vi "sv_Flat Pink Noise Filter Coefficients.vi"() -> (1 "pink noise coeffs out":T1[](array[typedef]) {"order" format="%#_6p"})   [LabVIEW 2017]
uses:
  <vilib>/addons/_NISVFA/_Generation/subVIs/sv_Flat Pink Noise Coefficients.ctl
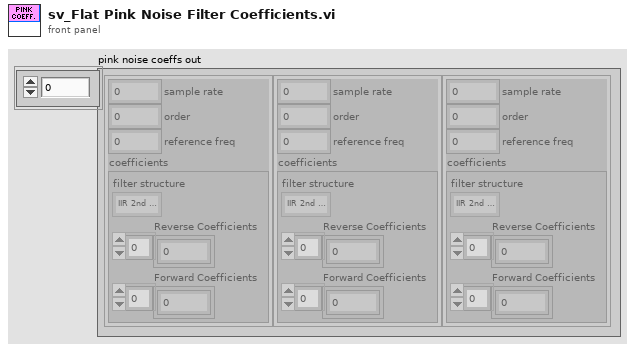
[diagram p1: front panel]
types:
  T1 = typedef "sv_Flat Pink Noise Coefficients.ctl" = cluster{"sample rate":dbl, "order":i32, "reference freq":dbl, "coefficients":cluster{"filter structure":enum32{"IIR 2nd Order", "IIR 4th Order"}, "Reverse Coefficients":dbl[], "Forward Coefficients":dbl[]}}
  T2 = cluster{"filter structure":enum32{"IIR 2nd Order", "IIR 4th Order"}, "b[i]":dbl[], "b[i]":dbl[]}
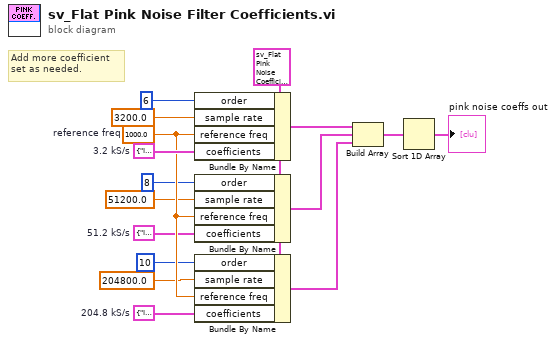
[diagram p0: block diagram]
diagram:
  w2 = T1 {"sample rate"=0.0, "order"=0, "reference freq"=0.0, "coefficients"={"filter structure"=enum."IIR 2nd Order", "Reverse Coefficients"=[-0.7577817918160894, 0.030536312542661648, -1.9301693255314603, 0.9308166907598192, -1.9976993495401576, 0.9976999449448676], "Forward Coefficients"=[1.0, -0.2630217874045446, -0.07790828981581392, 1.0, -1.8419617837757336, 0.8453487799874667, 1.0, -1.9944586178482333, 0.9944625262307424]}} ("pink noise filter coefficients")
  w13 = 1000.0  # reference freq
  w7 = T2 {"filter structure"=enum."IIR 2nd Order", "b[i]"=[-0.171965872867143, -0.14490435156532322, -1.8140302905202388, 0.8194425773674574, -1.9897817343295314, 0.989797517955009, -1.9994711490192336, 0.9994711911845989, -1.9999742046175086, 0.9999742047021241], "b[i]"=[1.0, 0.22536535952328549, -0.06368643558697416, 1.0, -1.6352135455544063, 0.6568002264131008, 1.0, -1.9786462720400246, 0.978715356715225, 1.0, -1.998890268418391, 0.9988904541594328, 1.0, -1.999943492291351, 0.9999434927563383]}  # 204.8 kS/s
  w8 = T2 {"filter structure"=enum."IIR 2nd Order", "b[i]"=[-0.4997415626209277, -0.0781165368933433, -1.899042766402168, 0.9004465196918887, -1.9961905976612995, 0.9961925515397482, -1.9998667384609488, 0.9998667405068554], "b[i]"=[1.0, -0.037290807411950844, -0.085296388532516, 1.0, -1.779133412098331, 0.7860409613819236, 1.0, -1.99129422933829, 0.9913044476118756, 1.0, -1.9996847928216734, 0.999684805808033]}  # 51.2 kS/s
  w16 = T2 {"filter structure"=enum."IIR 2nd Order", "b[i]"=[-0.7577817918160894, 0.030536312542661648, -1.9301693255314603, 0.9308166907598192, -1.9976993495401576, 0.9976999449448676], "b[i]"=[1.0, -0.2630217874045446, -0.07790828981581392, 1.0, -1.8419617837757336, 0.8453487799874667, 1.0, -1.9944586178482333, 0.9944625262307424]}  # 3.2 kS/s
  # "Add more coefficient\nset as needed."
  n1 = Bundle By Name(cluster=w2, "order"=6, "sample rate"=3200.0, "reference freq"=w13, "coefficients"=w16) -> (w6:T1)
  n2 = Bundle By Name(cluster=w2, "order"=8, "sample rate"=51200.0, "reference freq"=w13, "coefficients"=w8) -> (w5:T1)
  n3 = Bundle By Name(cluster=w2, "order"=10, "sample rate"=204800.0, "reference freq"=w13, "coefficients"=w7) -> (w4:T1)
  n4 = Build Array(w6, w5, w4) -> (w3:T1[])
  n5 = Sort 1D Array(array=w3) -> (sorted array=→"pink noise coeffs out":T1[])
